vi "MH_T2Interface.vi"() -> ()   [LabVIEW 2019]
panel:
  in  "Max T(s)":i32=1 min=1 max=10000 step=1
  in  "Show Avg":bool
  in  "Avg Val":i32=1 min=1 max=10000 step=1
  in  "Ch":enum16{"Ch1", "Ch2", "Ch3", "Ch4"}(ring)
  out "Data":cluster{"Max Val":dbl, "Curr.Val":dbl}
  in  "error in (no error)":errorcluster caption="entrée d'erreur (pas d'erreur)"
  out "Graph":T1(graph)
  out "error out":errorcluster caption="sortie d'erreur"
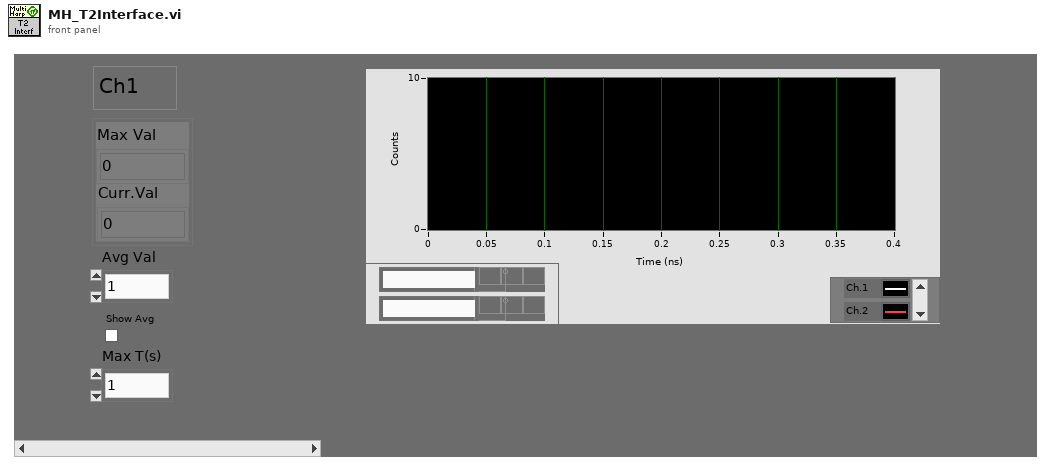
[diagram p1: front panel]
types:
  T1 = cluster{dbl, "Resolution (ns)":dbl, "Histogram":u32[][]}
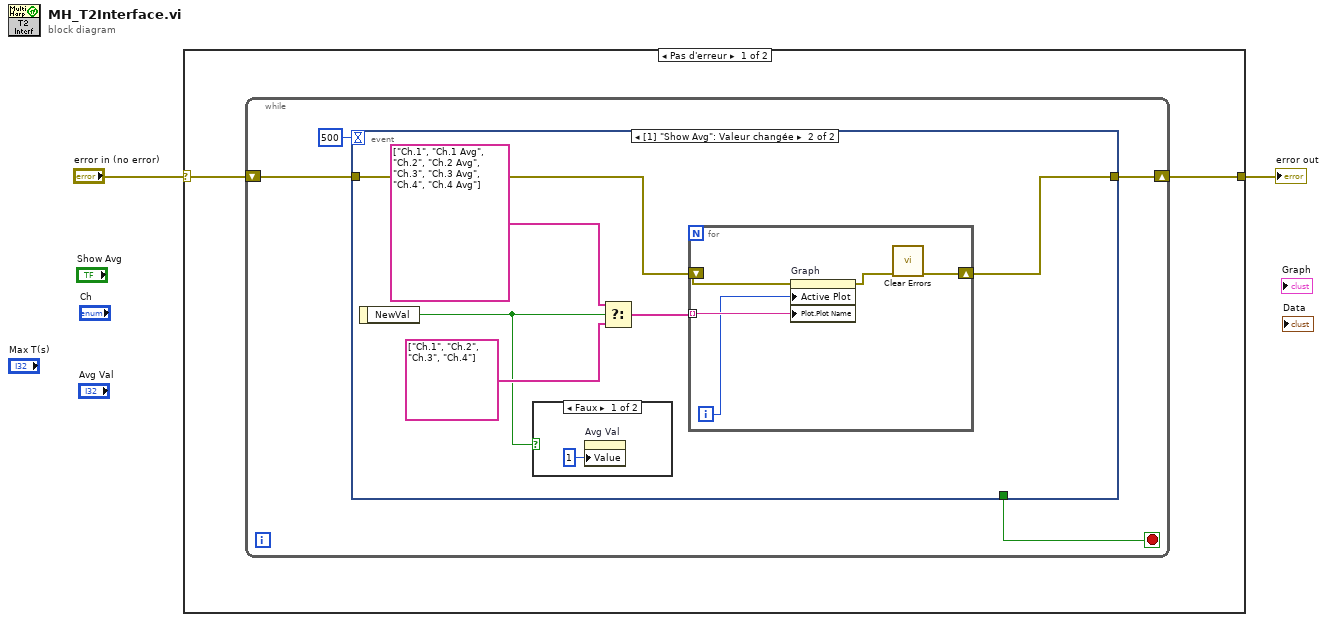
[diagram p0: block diagram]
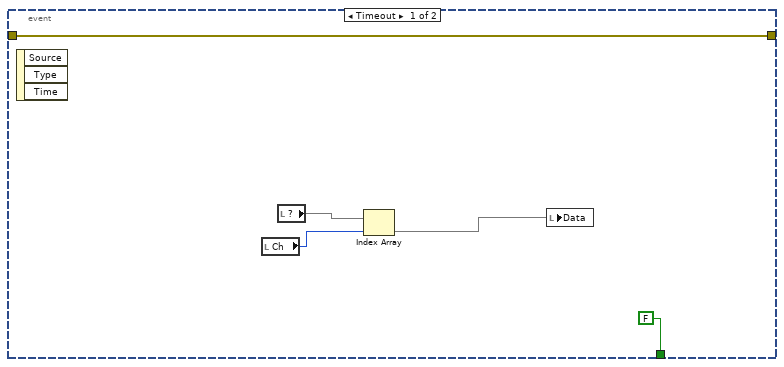
[diagram p2: hidden frame]
diagram:
  n1 = case shown="Pas d'erreur" "error in (no error)" {
    selector: "error in (no error)" -> [w3 w26]
    tunnel: [w4 w26] -> w2
    frame No Error {
      n2 = while {
        shift-right: [w7] -> w4
        shift-left: w3 -> [w6]
        stop <- w5 stop-if-true
        n3 = event shown="[1] \"Show Avg\": Valeur changée" {
          selector: _ -> [_ _]
          dyn-events: _ -> [_ _]
          timeout: 500 -> [_ _]
          tunnel: [w13 w15] -> w7
          tunnel: w6 -> [w13 w16]
          tunnel: [FALSE _] -> w5
          event Timeout {
            n4 = event-data() -> ()  [unwired: 1 in, 3 out]
            n5 = local read "Ch"() -> (w9:enum16{"Ch1", "Ch2", "Ch3", "Ch4"})
            n6 = local read item#-1() -> (w11)
            n7 = Index Array(array=w11, index=w9) -> (element=w10)
            n8 = local write "Data"(w10) -> ()
          }
          event "Show Avg": Value Change {
            n9 = event-data() -> ("NewVal"=w14:bool)  [unwired: 1 in]
            n10 = case shown="Faux" w14 {
              frame False {
                n11 = property on="Avg Val" class="NumNb (strict)"("Value"=1 ("Avg Val")) -> ()  [unwired: 2 in, 2 out]
              }
              frame True {
              }
            }
            n12 = Select(t=string[] ["Ch.1", "Ch.1 Avg", "Ch.2", "Ch.2 Avg", "Ch.3", "Ch.3 Avg", "Ch.4", "Ch.4 Avg"], s=w14, f=string[] ["Ch.1", "Ch.2", "Ch.3", "Ch.4"]) -> (s? t:f=w17:string[])
            n13 = for {
              tunnel: w17 -> [w25] mode=indexing
              shift-right: [w22] -> w15
              shift-left: w16 -> [w24]
              i -> [w21]
              n14 = property on="Graph" class="GraphWF (strict)"(error in=w24, "Active Plot"=w21, "Plot.Plot Name"=w25) -> (error out=w23:errorcluster)  [unwired: 1 in, 1 out]
              n15 = call <vilib>:"Clear Errors.vi"("error in (no error)"=w23) -> ("error out"=w22:errorcluster)  [unwired: 5 in, 1 out]
            }
          }
        }
      }
    }
    frame Error {
    }
  }
  "error out" <- w2
